vi "retrieve_vector.vi"(0 "vector_qdrant in":refnum<class "vector_qdrant.lvclass">, 5 "colection_name":string, 7 "id":string, 11 "error in (no error)":errorcluster) -> (4 "vector_qdrant out":refnum<class "vector_qdrant.lvclass">, 6 "vector":T1, 15 "error out":errorcluster)   [LabVIEW 2020, in "vector_qdrant.lvclass"]
uses:
  vector_qdrant.lvclass
  abstract_vector_base/vector.ctl
  vector_qdrant.lvclass/vector_qdrant.ctl
  <vilib>/httpClient/LabVIEWHTTPClient.lvlib
  abstract_vector_base/abstract_vector_base.lvclass
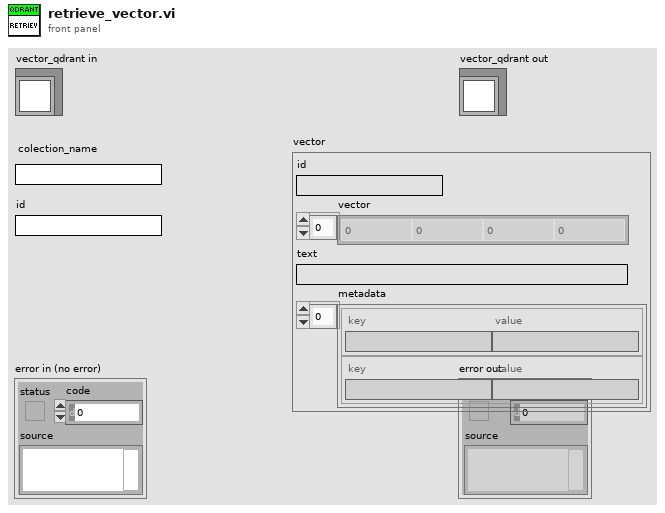
[diagram p1: front panel]
types:
  T1 = typedef "abstract_vector_base.lvclass/vector.ctl" = cluster{"id":string, "vector":dbl[], "text":string, "metadata":cluster{"key":string, "value":string}[]}
  T2 = typedef "LabVIEWHTTPClient.lvlib/ClientHandle.ctl" = refnum<k1>
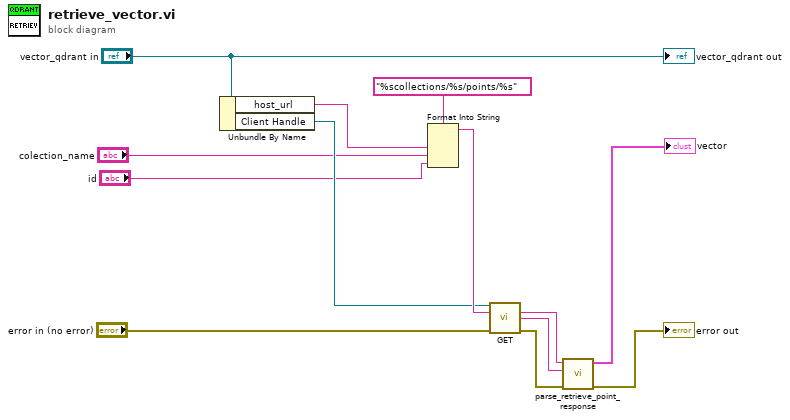
[diagram p0: block diagram]
diagram:
  n1 = Unbundle By Name("vector_qdrant in") -> ("host_url"=w8:string, "Client Handle"=w9:T2)
  n2 = Format Into String(format string="%scollections/%s/points/%s", w8, "colection_name", "id") -> (resulting string=w12:string)  [unwired: 2 in, 1 out]
  n3 = call <vilib>:"GET.vi"("client handle"=w9, "url"=w12, "error in (no error)"="error in (no error)") -> ("headers"=w5:string, "body"=w4:string, "error out"=w3:errorcluster)  [unwired: 9 in, 1 out]
  n4 = call "parse_retrieve_point_response.vi"("error in (no error)"=w3, "body"=w4, "headers"=w5) -> ("error out"=→"error out":errorcluster, "vector"=→"vector":T1)  [unwired: 7 in]
  "vector_qdrant out" <- "vector_qdrant in"
